vi "Actuator State Machine.vi"() -> ()   [LabVIEW 2012]
uses:
  Controls/Actuator Shifter.ctl
  Globals/Are We Calibrating Actuator.vi
  Globals/Autonomous Tipping.vi
  Globals/Potentiometers.vi
  <vilib>/Rock Robotics/WPI/Joystick/WPI_JoystickGetSetRefNum.vi
  Globals/Jaguar Commands.vi
  Globals/Max Tipper Angle.vi
panel:
  in  "Actuator Volt Limit":dbl=1.0
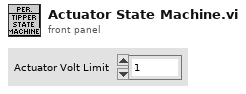
[diagram p1: front panel]
types:
  T1 = typedef "Actuator Shifter.ctl" = enum16{"Wait for Button", "Force Bridge Down", "Hold Bridge Down"}
  T2 = typedef "WPI_AnalogChannelDevRef.ctl" = cluster{"DevStatus":errorcluster, "Analog Module":T3, "Analog Channel":T4}
  T3 = typedef "FPGA_TypedefAnalogModule.ctl" = enum16{"Analog Module 1", "Analog Module 2"}
  T4 = typedef "FPGA_AIChannel.ctl" = enum8{"AI 1", "AI 2", "AI 3", "AI 4", "AI 5", "AI 6", "AI 7", "AI 8", "Invalid"}
  T5 = cluster{"Front Left":T2, "Front Right":T2, "Rear Left":T2, "Rear Right":T2, "Actuator":T2}
  T6 = typedef "WPI_JoystickDevRef.ctl" = cluster{"Device":T7}
  T7 = typedef "WPI_JoystickDeviceEnum.ctl" = enum16{"USB 1", "USB 2", "USB 3", "USB 4", "Kinect 1", "Kinect 2"}
  T8 = typedef "WPI_JoystickButtonState.ctl" = cluster{"Button 1":bool, "Button 2":bool, "Button 3":bool, "Button 4":bool, "Button 5":bool, "Button 6":bool, "Button 7":bool, "Button 8":bool, "Button 9":bool, "Button 10":bool, "Button 11":bool, "Button 12":bool}
  T9 = cluster{"axis 1 (x)":dbl, "axis 2 (y)":dbl, "axis 3 (throttle)":dbl, "axis 4":dbl, "axis 5":dbl, "axis 6":dbl}
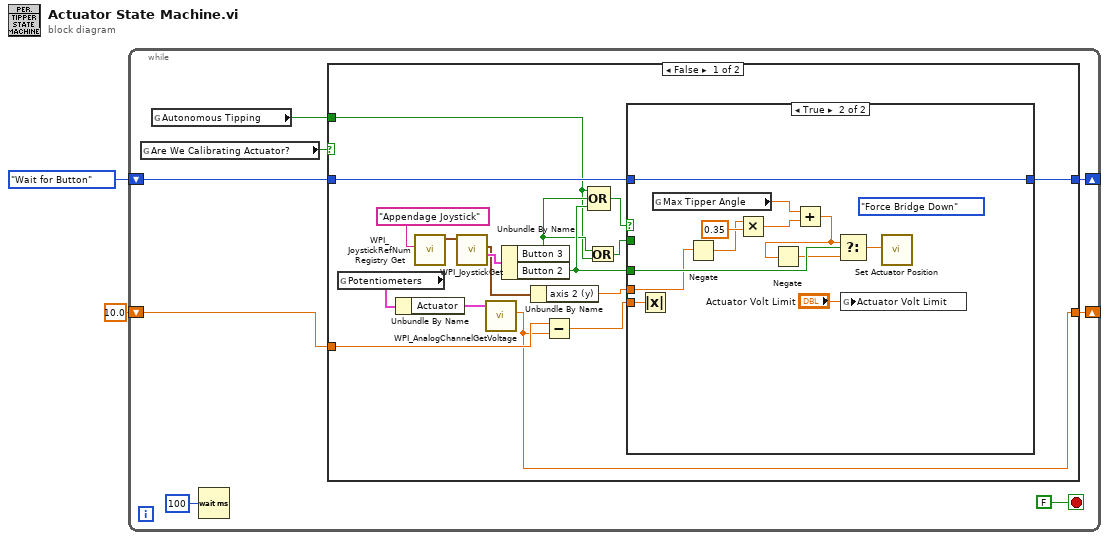
[diagram p0: block diagram]
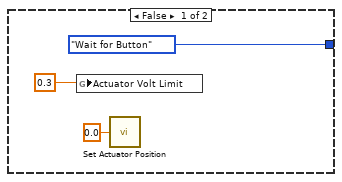
[diagram p2: hidden frame]
diagram:
  n1 = while {
    shift-right: [w8] -> _
    shift-left: 10.0 ("Voltage") -> [w7]
    shift-right: [w5] -> _
    shift-left: Actuator_Shifter."Wait for Button" -> [w4]
    stop <- FALSE stop-if-true
    n2 = global read "Are We Calibrating Actuator.vi" "Are We Calibrating Actuator?"() -> (w9:bool)
    n3 = global read "Autonomous Tipping.vi" "Autonomous Tipping"() -> (w3:bool)
    n4 = Wait (ms)(milliseconds to wait=u32 100) -> ()  [unwired: 1 out]
    n5 = case shown="False" w9 {
      tunnel: [w21 w44] -> w8
      tunnel: w7 -> [w22 w44]
      tunnel: [w20 w43] -> w5
      tunnel: w4 -> [w19 w43]
      tunnel: w3 -> [w13 _]
      frame False {
        n6 = global read "Potentiometers.vi" "Potentiometers"() -> (w24:T5)
        n7 = Unbundle By Name(w24) -> ("Actuator"=w23:T2)
        n8 = call <vilib>:"WPI_JoystickRefNum Registry Get.vi"("refnum name"="Appendage Joystick") -> ("JoystickDevRef"=w26:T6)  [unwired: 9 in, 1 out]
        n9 = call <vilib>:"WPI_JoystickGet.vi"("JoystickDevRef"=w26) -> ("Buttons"=w25:T8, "Axes"=w12:T9)  [unwired: 4 in, 1 out]
        n10 = call <vilib>:"WPI_AnalogChannelGetVoltage.vi"("AIDeviceRef"=w23) -> ("Voltage"=w21:dbl)  [unwired: 8 in, 2 out]
        n11 = Unbundle By Name(w25) -> ("Button 3"=w15:bool, "Button 2"=w16:bool)
        n12 = Unbundle By Name(w12) -> ("axis 2 (y)"=w11:dbl)
        n13 = Subtract(x=w22, y=w21) -> (x-y=w18:dbl)
        n14 = Compound Arithmetic op=OR(w13, w15, w16) -> (w17:bool)
        n15 = Or(x=w15, y=w13) -> (x .or. y?=w14:bool)
        n16 = case shown="True" w17 {
          tunnel: w18 -> [_ w42]
          tunnel: [Actuator_Shifter."Wait for Button" w41] -> w20
          tunnel: w19 -> [_ w41]
          tunnel: w16 -> [_ w40]
          tunnel: w14 -> [_ _]
          tunnel: w11 -> [_ w34]
          frame False {
            n17 = global write "Jaguar Commands.vi" "Actuator Volt Limit"(0.3 ("Actuator Volt Limit")) -> ()
            n18 = call "Set Actuator Position.vi"("Setpoint from Home"=0.0) -> ()
          }
          frame True {
            (unwired) Actuator_Shifter."Force Bridge Down"
            n19 = Absolute Value(x=w42) -> ()  [unwired: 1 out]
            n20 = global read "Max Tipper Angle.vi" "Max Tipper Angle"() -> (w37:dbl)
            n21 = Negate(x=w34) -> (-x=w32:dbl)
            n22 = Multiply(x=w32, y=0.35) -> (x*y=w31:dbl)
            n23 = Add(x=w37, y=w31) -> (x+y=w35:dbl)
            n24 = Negate(x=w35) -> (-x=w36:dbl)
            n25 = Select(t=w35, s=w40, f=w36) -> (s? t:f=w38:dbl)
            n26 = global write "Jaguar Commands.vi" "Actuator Volt Limit"("Actuator Volt Limit") -> ()
            n27 = call "Set Actuator Position.vi"("Setpoint from Home"=w38) -> ()
          }
        }
      }
      frame True {
      }
    }
  }
